vi "GetLastCompatibleVersion.vi"(8 "error in (no error)":errorcluster, 11 "LabVIEW Object":refnum<class>) -> (0 "error out":errorcluster, 2 "Last Compatible Class Version":T3, 3 "Current Class Version":T3)   [LabVIEW 2019, in "BlueSerialization.lvlib" / "BlueSerializer.lvclass"]
uses:
  BlueSerializer.lvclass
  <vilib>/Utility/EditLVLibs/LibVersion.ctl
  <vilib>/Utility/EditLVLibs/LVClass/Mutation History.ctl
  <vilib>/Utility/EditLVLibs/LVClass/Mutation Record.ctl
  <vilib>/Utility/EditLVLibs/Edit LVLibs.lvlib
panel:
  out "Mutation History":T1 {"LabVIEW Version" format="%.0x"}
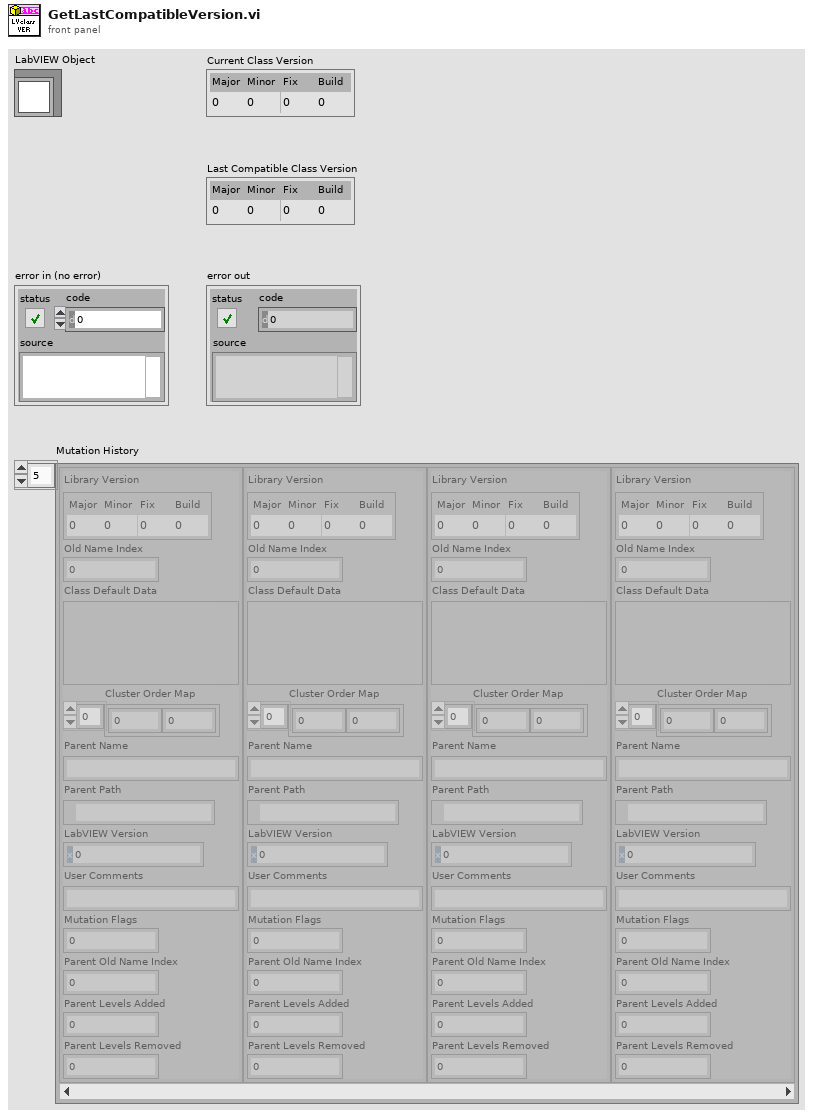
[diagram p1: front panel]
types:
  T1 = typedef "Edit LVLibs.lvlib/Mutation History.ctl" = T2[]
  T2 = typedef "Edit LVLibs.lvlib/Mutation Record.ctl" = cluster{"Library Version":T3, "Old Name Index":u8, "Class Default Data":variant, "Cluster Order Map":u32[], "Parent Name":string, "Parent Path":path, "LabVIEW Version":u32, "User Comments":string, "Mutation Flags":u8, "Parent Old Name Index":u8, "Parent Levels Added":u16, "Parent Levels Removed":u16}
  T3 = typedef "Edit LVLibs.lvlib/LibVersion.ctl" = cluster{"Major":u16, "Minor":u16, "Fix":u16, "Build":u16}
  T4 = cluster{"Major":u16, "Old Name Index":u8, "Parent Old Name Index":u8, "Parent Levels Added":u16, "Parent Levels Removed":u16}
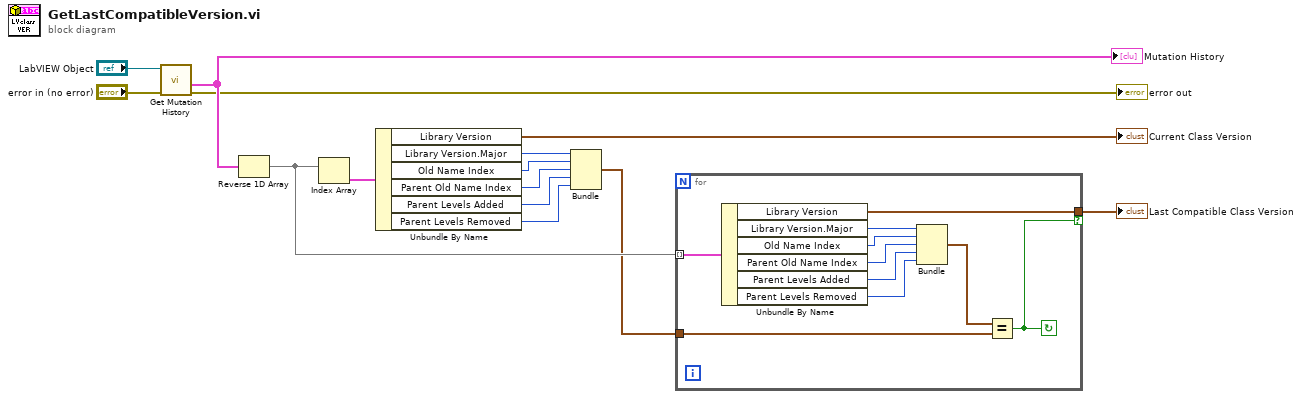
[diagram p0: block diagram]
diagram:
  n1 = call <vilib>:"Get Mutation History.vi"("error in"="error in (no error)", "Input object"="LabVIEW Object") -> ("error out"=→"error out":errorcluster, "Mutation History"=w4:T1)  [unwired: 6 in]
  "Mutation History" <- w4
  n2 = Reverse 1D Array(array=w4) -> (reversed array=w5:T1)
  n3 = Index Array(array=w5) -> (element=w12:T2)  [unwired: 1 in]
  n4 = Unbundle By Name(w12) -> ("Library Version"=→"Current Class Version":T3, "Library Version.Major"=w10:u16, "Old Name Index"=w9:u8, "Parent Old Name Index"=w8:u8, "Parent Levels Added"=w7:u16, "Parent Levels Removed"=w6:u16)
  n5 = Bundle("Major"=w10, "Old Name Index"=w9, "Parent Old Name Index"=w8, "Parent Levels Added"=w7, "Parent Levels Removed"=w6) -> (w3:T4)  [unwired: 1 in]
  n6 = for {
    tunnel: w5 -> [w19] mode=indexing
    tunnel: [w18] -> w2 if=w15
    tunnel: w3 -> [w16]
    stop <- w15 continue-if-true
    n7 = Unbundle By Name(w19) -> ("Library Version"=w18:T3, "Library Version.Major"=w20:u16, "Old Name Index"=w21:u8, "Parent Old Name Index"=w22:u8, "Parent Levels Added"=w23:u16, "Parent Levels Removed"=w24:u16)
    n8 = Bundle("Major"=w20, "Old Name Index"=w21, "Parent Old Name Index"=w22, "Parent Levels Added"=w23, "Parent Levels Removed"=w24) -> (w17:T4)  [unwired: 1 in]
    n9 = Equal?(x=w17, y=w16) -> (x = y?=w15:bool)
  }
  "Last Compatible Class Version" <- w2
